vi "Write Display mode.vi"(8 "error in (no error)":errorcluster, 10 "Display mode":T1, 11 "U32 D Element in":refnum<class "U32 D Element.lvclass">) -> (0 "error out":errorcluster, 3 "U32 D Element out":refnum<class "U32 D Element.lvclass">)   [LabVIEW 2018, in "D Datagrid Library.lvlib" / "U32 D Element.lvclass"]
uses:
  U32 D Element.lvclass
  Display mode.ctl
  U32 D Element.lvclass/U32 D Element.ctl
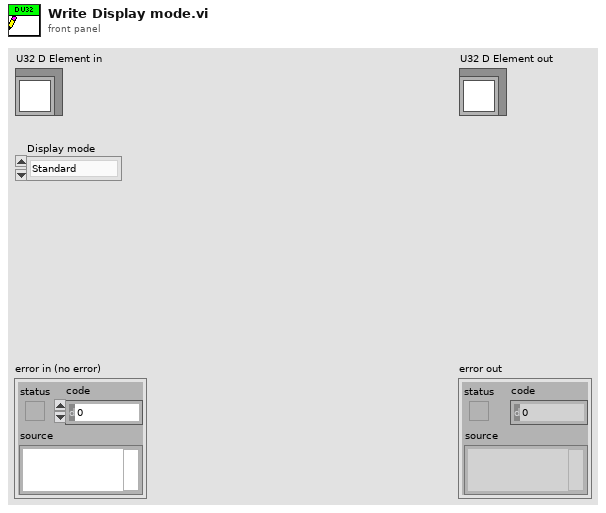
[diagram p1: front panel]
types:
  T1 = typedef "D Datagrid Library.lvlib/U32 D Element.lvclass/Display mode.ctl" = enum16{"Standard", "Hex"}
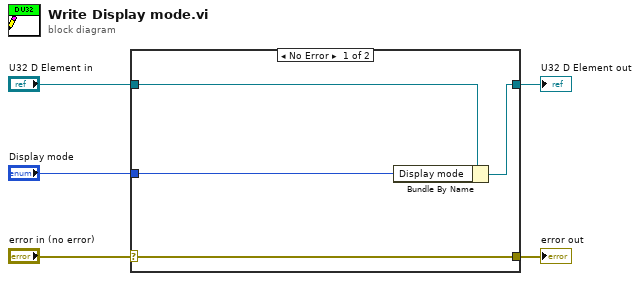
[diagram p0: block diagram]
diagram:
  n1 = case shown="No Error" "error in (no error)" {
    selector: "error in (no error)" -> [w9 w10]
    tunnel: [w9 w10] -> w4
    tunnel: [w7 w11] -> w2
    tunnel: "U32 D Element in" -> [w8 w11]
    tunnel: "Display mode" -> [w6 _]
    frame No Error {
      n2 = Bundle By Name(cluster=w8, "Display mode"=w6) -> (w7:refnum<class "U32 D Element.lvclass">)
    }
    frame Error {
    }
  }
  "error out" <- w4
  "U32 D Element out" <- w2
